vi "Render Sidebar Text.vi"(7 "Renderer":refnum<class "Renderer.lvclass">, 8 "error in (no error)":errorcluster, 11 "Ship in":refnum<class "Ship.lvclass">) -> (0 "error out":errorcluster)   [LabVIEW 2021, in "Ship.lvclass"]
uses:
  Ship.lvclass
  Renderer/Renderer.lvclass
  Ship.lvclass/Ship.ctl
  Re-use Libraries/Vector 2D/Vector 2D.lvclass
  LabSDL2/Source/Libraries/SDL2 Utility/Point (I32).ctl
  LabSDL2/Source/Libraries/SDL2 Utility/SDL2 Utility.lvlib
  Resource Manager/Resource Manager.lvclass
  Texture/Texture.lvclass
  Element/Element.lvclass
  Math/Math.lvlib
panel:
  in  "Race":i32=10
  in  "Captain":i32=210
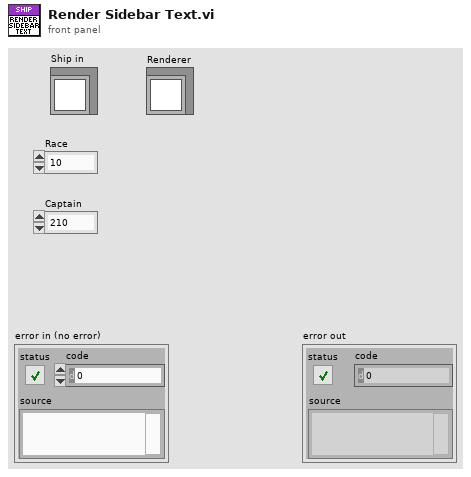
[diagram p1: front panel]
types:
  T1 = typedef "SDL2 Utility.lvlib/Point (I32).ctl" = cluster{"x":i32, "y":i32}
  T2 = typedef "Constants.ctl" = cluster{"Colours":cluster{"OK":u32, "Warning":u32, "Error":u32, "Red":u32, "Green":u32, "Blue":u32, "Yellow":u32}, "System":cluster{"Target Frames Second":dbl, "World Size":T1, "Window Size":T1, "Battle Area Size":T1, "Sidebar Scaling":sgl, "Sidebar Width":i32, "SC2 Frame Rate [Seconds/Frame]":sgl}, "Game":cluster{"Maximum Asteroids":i32, "Max Energy":i32, "Max Crew":i32, "Maximum Stars":i32}}
  T3 = typedef "Element.lvclass/Player Type.ctl" = enum16{"Neutral", "Player 1", "Player 2"}
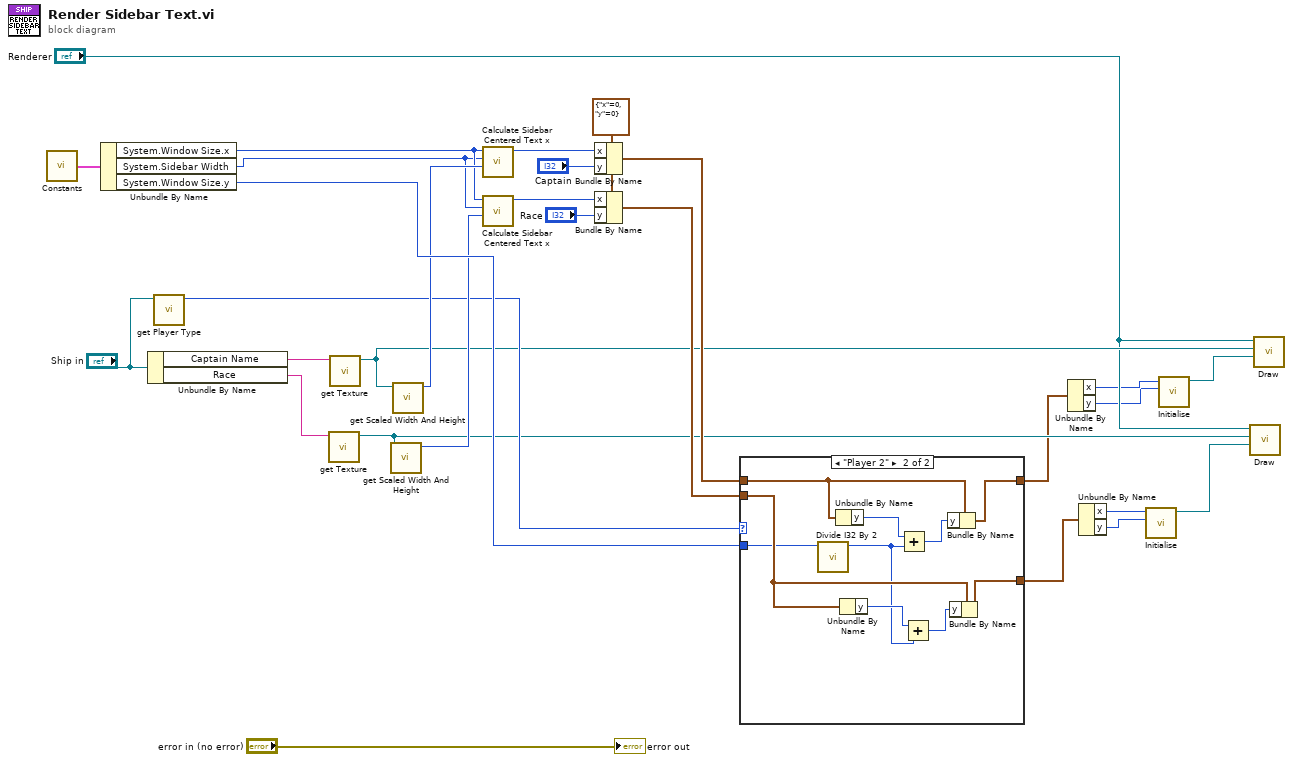
[diagram p0: block diagram]
diagram:
  w18 = T1 {"x"=0, "y"=0} ("Icon Offsets")
  n1 = call "Constants.vi"() -> ("Constants"=w28:T2)
  n2 = Unbundle By Name(w28) -> ("System.Window Size.x"=w21:i32, "System.Sidebar Width"=w20:i32, "System.Window Size.y"=w27:i32)
  n3 = Unbundle By Name("Ship in") -> ("Captain Name"=w26:string, "Race"=w22:string)
  n4 = call "get Player Type.vi"("Element in"="Ship in") -> ("Player Type"=w13:T3)  [unwired: 10 in]
  n5 = call "get Texture.vi"("Texture Name"=w22) -> ("Texture"=w9:refnum<class "Texture.lvclass">)  [unwired: 10 in]
  n6 = call "get Texture.vi"("Texture Name"=w26) -> ("Texture"=w11:refnum<class "Texture.lvclass">)  [unwired: 10 in]
  n7 = call "get Scaled Width And Height.vi"("Texture in"=w9) -> ("Width"=w19:i32)  [unwired: 9 in, 1 out]
  n8 = call "get Scaled Width And Height.vi"("Texture in"=w11) -> ("Width"=w24:i32)  [unwired: 9 in, 1 out]
  n9 = call "Calculate Sidebar Centered Text x.vi"("Width"=w24, "Sidebar Width"=w20, "x"=w21) -> ("Numeric"=w23:i32)  [unwired: 8 in]
  n10 = call "Calculate Sidebar Centered Text x.vi"("Width"=w19, "Sidebar Width"=w20, "x"=w21) -> ("Numeric"=w16:i32)  [unwired: 8 in]
  n11 = Bundle By Name(cluster=w18, "x"=w23, "y"="Captain") -> (w25:T1)
  n12 = Bundle By Name(cluster=w18, "x"=w16, "y"="Race") -> (w17:T1)
  n13 = case shown="\"Player 2\"" w13 {
    tunnel: w25 -> [w31 w41]
    tunnel: [w31 w38] -> w7
    tunnel: w27 -> [_ w33]
    tunnel: w17 -> [w30 w35]
    tunnel: [w30 w34] -> w4
    frame "Player 1", Default {
    }
    frame "Player 2" {
      n14 = call "Divide I32 By 2.vi"("Value"=w33) -> ("Value/2"=w32:i32)  [unwired: 10 in]
      n15 = Unbundle By Name(w41) -> ("y"=w40:i32)
      n16 = Unbundle By Name(w35) -> ("y"=w36:i32)
      n17 = Add(x=w40, y=w32) -> (x+y=w39:i32)
      n18 = Add(x=w36, y=w32) -> (x+y=w37:i32)
      n19 = Bundle By Name(cluster=w41, "y"=w39) -> (w38:T1)
      n20 = Bundle By Name(cluster=w35, "y"=w37) -> (w34:T1)
    }
  }
  n21 = Unbundle By Name(w7) -> ("x"=w6:i32, "y"=w5:i32)
  n22 = Unbundle By Name(w4) -> ("x"=w3:i32, "y"=w2:i32)
  n23 = call "Initialise.vi"("y"=w2, "x"=w3) -> ("Vector 2D out"=w1:refnum<class "Vector 2D.lvclass">)  [unwired: 9 in]
  n24 = call "Initialise.vi"("y"=w5, "x"=w6) -> ("Vector 2D out"=w8:refnum<class "Vector 2D.lvclass">)  [unwired: 9 in]
  n25 = call "Draw.vi"("Destination"=w1, "Texture"=w9, "Renderer"="Renderer") -> ()  [unwired: 8 in, 1 out]
  n26 = call "Draw.vi"("Destination"=w8, "Texture"=w11, "Renderer"="Renderer") -> ()  [unwired: 8 in, 1 out]
  "error out" <- "error in (no error)"
